vi "Destroy Client.vi"(8 "error in (no error)":errorcluster, 11 "Json Logger in":refnum<class "Json Logger.lvclass">) -> (0 "error out":errorcluster, 3 "Json Logger out":refnum<class "Json Logger.lvclass">)   [LabVIEW 2021, in "Json Logger.lvclass"]
uses:
  Json Logger.lvclass
  Json Logger.lvclass/Json Logger.ctl
  log_measurement_client/log_measurement_client.lvlib
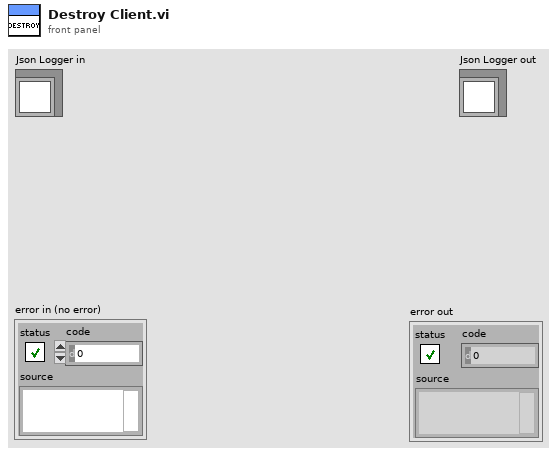
[diagram p1: front panel]
types:
  T1 = typedef "grpc-lvsupport-release.lvlib/grpcId.ctl" = u64
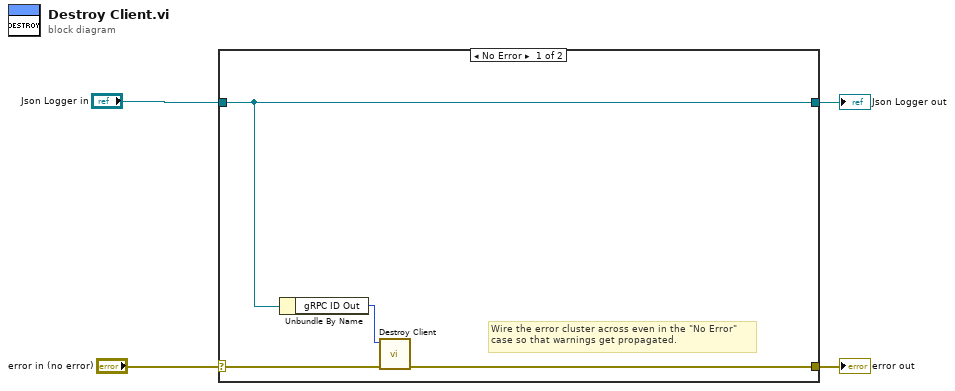
[diagram p0: block diagram]
diagram:
  n1 = case shown="No Error" "error in (no error)" {
    selector: "error in (no error)" -> [w8 w10]
    tunnel: [w7 w10] -> w3
    tunnel: "Json Logger in" -> [w5 w9]
    tunnel: [w5 w9] -> w1
    frame No Error {
      # "Wire the error cluster across even in the \"No Error\"\ncase so that warnings get propagated."
      n2 = Unbundle By Name(w5) -> ("gRPC ID Out"=w6:T1)
      n3 = call "Destroy Client.vi"("error in"=w8, "gRPC ID"=w6) -> ("error out"=w7:errorcluster)  [unwired: 9 in]
    }
    frame Error {
    }
  }
  "error out" <- w3
  "Json Logger out" <- w1
